vi "2021_day3_task1.vi"() -> ()   [LabVIEW 2021]
panel:
  out "x*y":u32
  out "Epsilon (DEC)":u32
  out "Gamma (DEC)":u32
  out "GAMA":bool[](array[boolean])
  out "EPSILON":bool[](array[boolean])
  out "size(s)":i32
  out "Array 2":i32[](array[numeric])
  out "Array":i32[][](array[numeric])
  out "array 2":string[](array[string])
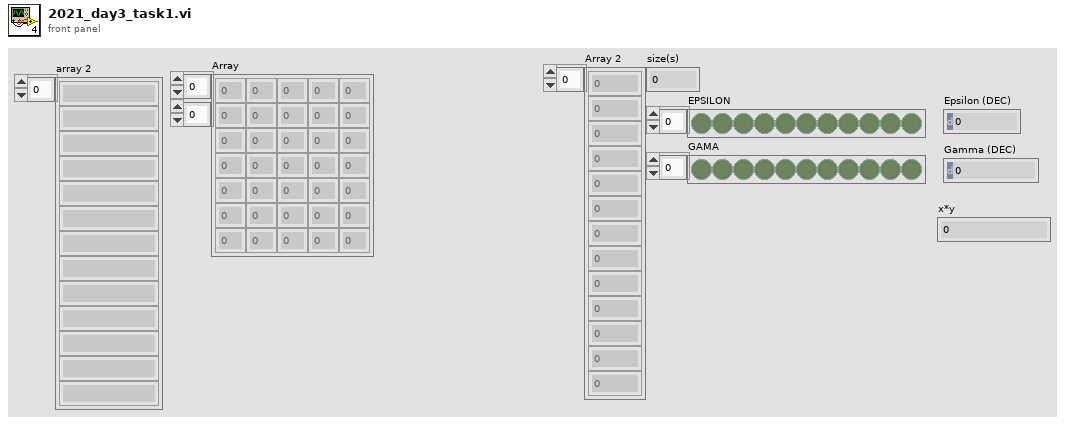
[diagram p1: front panel]
diagram:
  (unwired) "00100\n11110\n10110\n10111\n10101\n01111\n00111\n11100\n10000\n11001\n00010\n01010"
  n1 = Spreadsheet String To Array(delimiter (Tab)="\n", format string="%s", spreadsheet string="000111111001\n111011110110\n101111111000\n111100100110\n001111011000\n011100010110\n000101001001\n100001100101\n000011111100\n110000101000\n011110110101\n011000111100\n011000001011\n010111101101\n011111100010\n100110001111\n100111100100\n111110010100\n101001001110\n110101111110\n110110100000\n001010001110\n101100001100\n111001011000\n100101111111\n001001010100\n100111011000\n100101100000\n010001010101\n000111001100\n001100011110\n101100010101\n111011000011\n010000001110\n110000000110\n001010110000\n100011001111\n110100111101\n111111010100\n000101110111\n011110101111\n100110000110\n010011000000\n000110010000\n101101101011\n011101100011\n01...", array type (2D Dbl)=string[] []) -> (array=w12:string[])
  "array 2" <- w12
  n2 = for {
    tunnel: w12 -> [w21] mode=indexing
    tunnel: [w19] -> w15 mode=indexing
    n3 = String Length(string=w21) -> (length=w22:i32)
    n4 = for {
      N: w22 -> [_]
      shift-right: [w25] -> _
      shift-left: w21 -> [w25]
      tunnel: [w23] -> w20 mode=indexing
      i -> [w24]
      n5 = String Subset(string=w25, offset (0)=w24, length (rest)=1 ("length (rest)")) -> (substring=w23:string)
    }
    n6 = Decimal String To Number(string=w20) -> (number=w19:i32[])  [unwired: 2 in, 1 out]
  }
  "Array" <- w15
  n7 = Array Size(array=w12) -> (size(s)=w11:i32)
  "size(s)" <- w11
  n8 = Divide(x=w11, y=2) -> (x/y=w10:dbl)
  n9 = Transpose 2D Array(2D array=w15) -> (transposed array=w14:i32[][])
  n10 = for {
    tunnel: w14 -> [w30] mode=indexing
    tunnel: [w29] -> w13 mode=indexing
    tunnel: w10 -> [w28]
    tunnel: [w27] -> w8 mode=indexing
    n11 = Add Array Elements(numeric array=w30) -> (sum=w29:i32)
    n12 = Greater?(x=w28, y=w29) -> (0:w27:bool)
  }
  "Array 2" <- w13
  "EPSILON" <- w8
  n13 = Not(x=w8) -> (.not. x?=w7:bool[])
  "GAMA" <- w7
  n14 = Reverse 1D Array(array=w8) -> (reversed array=w5:bool[])
  n15 = Reverse 1D Array(array=w7) -> (reversed array=w6:bool[])
  n16 = Boolean Array To Number(Boolean array=w6) -> (number=w4:u32)
  "Gamma (DEC)" <- w4
  n17 = Boolean Array To Number(Boolean array=w5) -> (number=w3:u32)
  "Epsilon (DEC)" <- w3
  n18 = Multiply(x=w4, y=w3) -> (x*y=→"x*y":u32)
